vi "Pre Launch Init.vi"(11 "CS++Scope in":refnum<class "CS++Scope.lvclass">) -> (0 "error out":errorcluster, 3 "CS++Scope out":refnum<class "CS++Scope.lvclass">)   [LabVIEW 2013, in "CS++Scope.lvlib" / "CS++Scope.lvclass"]
doc: "(<B>Filename</B>: Actor Framework.lvlib:Actor.lvclass:Pre Launch Init.vi)\n\nDefines behavior that occurs after the Launch Actor method is invoked but before the actor's Actor Core method begins running.\n\nThe Pre Launch Init method is guaranteed to finish before the Launch Actor method returns to its caller and before the actor itself receives any messages. Any references that the Pre Launch Init method obtains are guaranteed to have the same lifetime as the actor itself. Any errors that the Pre Launch Init method returns will abort the launch.\n\nBy default, this method does nothing. A descendant class may override it to define behavior."
uses:
  CS++Scope.lvclass
  CSPP_Core/Actors/CS++DeviceActor/CS++DeviceActor.lvclass
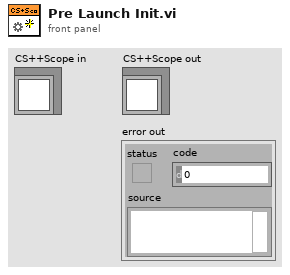
[diagram p1: front panel]
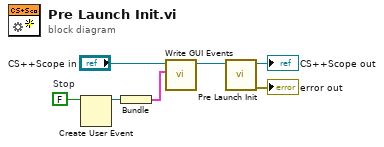
[diagram p0: block diagram]
diagram:
  w1 = FALSE  # Stop
  n1 = Create User Event(user event datatype=w1) -> (user event=w2:refnum<user-event>)  [unwired: 1 in, 1 out]
  n2 = Bundle("Stop"=w2) -> (w3:cluster{"Stop":refnum<user-event>})  [unwired: 1 in]
  n3 = call-dynamic "Write GUI Events.vi"("GUI Events"=w3, "CS++Scope in"="CS++Scope in") -> ("CS++Scope out"=w4:refnum<class "CS++Scope.lvclass">)  [unwired: 8 in, 1 out]
  n4 = call-parent "Pre Launch Init.vi"("CS++DeviceActor in"=w4) -> ("error out"=→"error out":errorcluster, "CS++DeviceActor out"=→"CS++Scope out":refnum<class "CS++Scope.lvclass">)  [unwired: 9 in]
